vi "FGV_Timer.vi"(7 "State":T1, 10 "error in (no error)":errorcluster, 11 "Set Time":i32) -> (2 "error out":errorcluster, 3 "Elapsed Time":dbl, 5 "Elapsed ?":bool)   [LabVIEW 2019]
uses:
  Typedef/Timer State.ctl
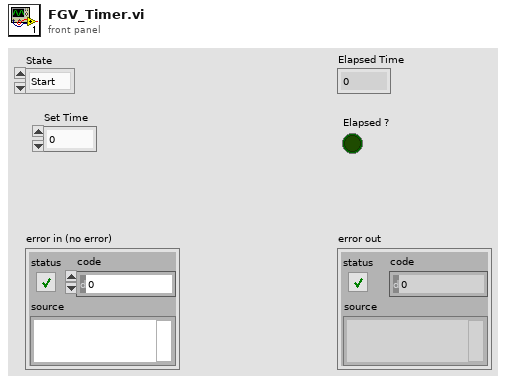
[diagram p1: front panel]
types:
  T1 = typedef "Timer State.ctl" = enum16{"Start", "Check"}
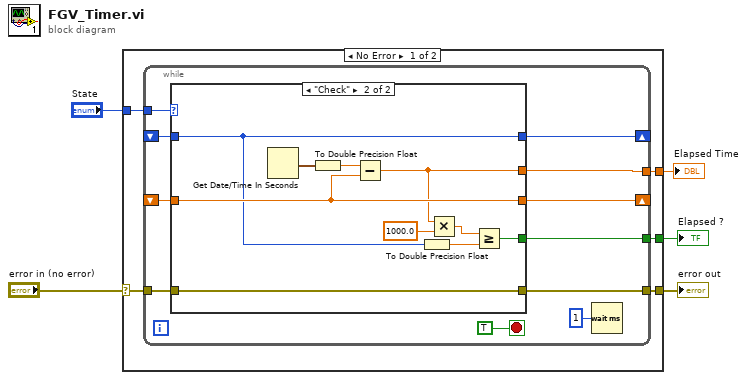
[diagram p0: block diagram]
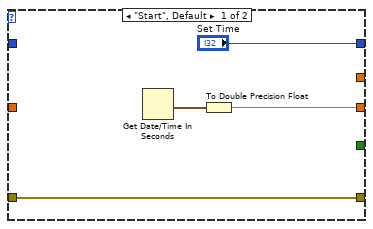
[diagram p2: hidden frame]
diagram:
  n1 = case shown="No Error" "error in (no error)" {
    selector: "error in (no error)" -> [w8 w36]
    tunnel: "State" -> [w10 _]
    tunnel: [w9 _] -> w4
    tunnel: [w7 w36] -> w2
    tunnel: [w6 _] -> w1
    frame No Error {
      n2 = while {
        tunnel: w10 -> [w21]
        shift-right: [w20] -> _
        shift-left: _ -> [w19]
        tunnel: [w17] -> w9
        tunnel: w8 -> [w16]
        tunnel: [w15] -> w7
        shift-right: [w13] -> _
        shift-left: _ -> [w12]
        tunnel: [w11] -> w6
        stop <- TRUE stop-if-true
        n3 = case shown="\"Check\"" w21 {
          tunnel: [w24 w33] -> w20
          tunnel: w19 -> [_ w33]
          tunnel: [_ w30] -> w17
          tunnel: w16 -> [w23 w32]
          tunnel: [w23 w32] -> w15
          tunnel: ["Set Time" w28] -> w13
          tunnel: w12 -> [_ w28]
          tunnel: [_ w26] -> w11
          frame "Start", Default {
            n4 = Get Date/Time In Seconds() -> (seconds since 1Jan1904=w25:timestamp)
            n5 = To Double Precision Float(number=w25) -> (double precision float=w24:dbl)
          }
          frame "Check" {
            n6 = Get Date/Time In Seconds() -> (seconds since 1Jan1904=w35:timestamp)
            n7 = To Double Precision Float(number=w35) -> (double precision float=w34:dbl)
            n8 = Subtract(x=w34, y=w33) -> (x-y=w30:dbl)
            n9 = To Double Precision Float(number=w28) -> (double precision float=w27:dbl)
            n10 = Multiply(x=w30, y=1000.0) -> (x*y=w31:dbl)
            n11 = Greater Or Equal?(x=w31, y=w27) -> (x >= y?=w26:bool)
          }
        }
        n12 = Wait (ms)(milliseconds to wait=u32 1) -> ()  [unwired: 1 out]
      }
    }
    frame Error {
    }
  }
  "Elapsed Time" <- w4
  "error out" <- w2
  "Elapsed ?" <- w1
